vi "DAQmx Create Channel (AI-Position-RVDT).vi"(0 "task in":refnum<k21>, 1 "maximum value":dbl=70.0 format="%0.2f", 2 "minimum value":dbl=-70.0 format="%0.2f", 3 "voltage excitation wire mode":i32(ring)=4 items=["4-Wire"=4, "5-Wire"=5], 5 "physical channels":tag, 6 "voltage excitation source":i32(ring)=10200 items=["Internal"=10200, "External"=10167, "None"=10230], 7 "name to assign":string, 8 "voltage excitation value":dbl=1.0, 9 "units":i32(ring)=10146 items=["Degrees"=10146, "Radians"=10273, "From Custom Scale"=10065], 10 "voltage excitation frequency":dbl=2500.0, 11 "error in":errorcluster, 12 "custom scale name":tag, 13 "sensitivity":dbl=50.0, 14 "sensitivity units":i32(ring)=12507 items=["mVolts/Volt/Degree"=12507, "mVolts/Volt/Radian"=12508]) -> (4 "task out":refnum<k21>, 15 "error out":errorcluster)   [LabVIEW 2011]
doc: "Creates channel(s) that use an RVDT to measure angular position."
uses:
  C:/Program Files/National Instruments/LabVIEW 2011/resource/objmgr/daqmx.rc
panel:
  # "input limits"
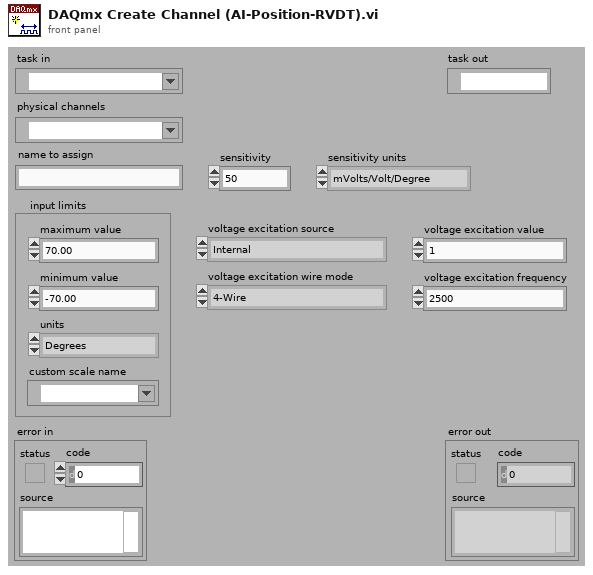
[diagram p1: front panel]
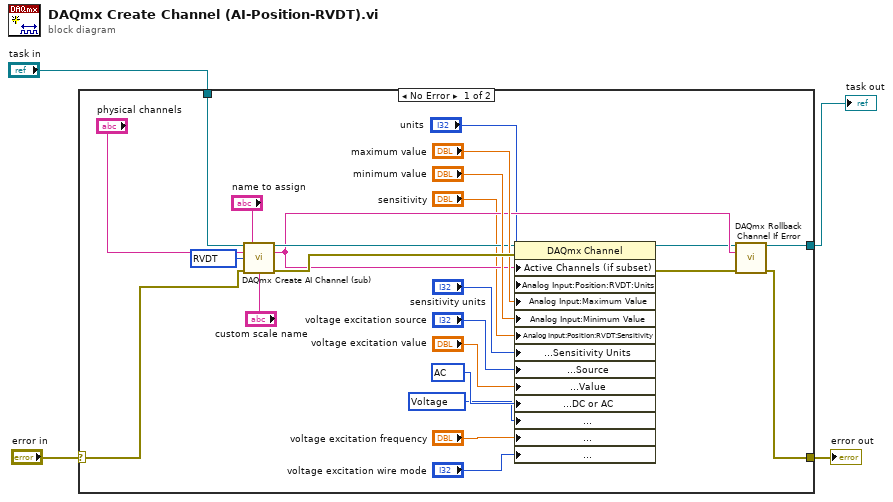
[diagram p0: block diagram]
diagram:
  n1 = case shown="No Error" "error in" {
    selector: "error in" -> [w27 w30]
    tunnel: [w18 w30] -> w2
    tunnel: "task in" -> [w28 w29]
    tunnel: [w19 w29] -> w1
    frame No Error {
      w5 = 10322 items=["Voltage"=10322, "Current"=10134] ("AI.Excit.VoltageOrCurrent")
      w6 = 10045 items=["DC"=10050, "AC"=10045] ("AI.Excit.DCorAC")
      w9 = 10353 items=["Voltage"=10322, "Current"=10134, "More:Voltage:Custom with Excitation"=10323, "More:Current:Custom with Excitation"=10136, "Frequency"=10181, "Period"=10257, "Resistance"=10278, "Temperature:Thermocouple"=10303, "Temperature:Thermistor"=10302, "Temperature:RTD"=10301, "Temperature:Built-in Sensor"=10311, "Strain Gage"=10300, "LVDT"=10352, "RVDT"=10353, "Accelerometer:Voltage Input"=10355, "Accelerometer:Current Input"=10356] ("measurement type")
      n2 = call "DAQmx Create AI Channel (sub).vi"("task in"=w28, "virtual channel name"="name to assign", "physical channel name"="physical channels", "measurement type"=w9, "error in"=w27, "custom scale"="custom scale name") -> ("task out"=w20:refnum<k21>, "channel names"=w17:string, "error out"=w24:errorcluster)  [unwired: 1 in, 6 out]
      n3 = property class="DAQmx Channel"(reference=w20, error in=w24, "Active Channels (if subset)"=w17, "Analog Input:Position:RVDT:Units"="units", "Analog Input:Maximum Value"="maximum value", "Analog Input:Minimum Value"="minimum value", "Analog Input:Position:RVDT:Sensitivity"="sensitivity", "Analog Input:Position:RVDT:Sensitivity Units"="sensitivity units", "Analog Input:General Properties:Signal Conditioning:Excitation:Source"="voltage excitation source", "Analog Input:General Properties:Signal Conditioning:Excitation:Value"="voltage excitation value", "Analog Input:General Properties:Signal Conditioning:Excitation:Advanced:DC or AC"=w6, "Analog Input:General Properties:Signal Conditioning:Excitation:Advanced:Voltage or Current"=w5, "Analog Input:General Properties:Signal Conditioning:Excitation:AC Excitation:Frequency"="voltage excitation frequency", "Analog Input:General Properties:Signal Conditioning:Excitation:AC Excitation:Wire Mode"="voltage excitation wire mode") -> (reference out=w16:refnum<k21>, error out=w15:errorcluster)
      n4 = call "DAQmx Rollback Channel If Error.vi"("task in"=w16, "channel names"=w17, "error in"=w15) -> ("task out"=w19:refnum<k21>, "error out"=w18:errorcluster)  [unwired: 11 out]
    }
    frame Error {
    }
  }
  "error out" <- w2
  "task out" <- w1
